vi "FFD.vi"(1 "CK":bool, 2 "Data":bool) -> (0 "Data 2":bool)   [LabVIEW 2012]
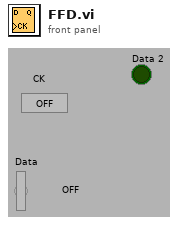
[diagram p1: front panel]
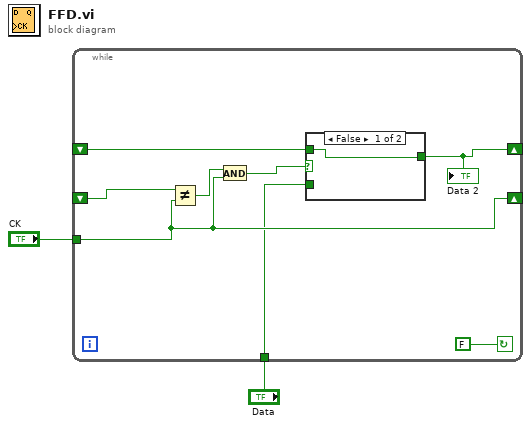
[diagram p0: block diagram]
diagram:
  n1 = while {
    shift-right: [w4] -> _
    shift-left: _ -> [w10]
    shift-right: [w7] -> _
    shift-left: _ -> [w6]
    tunnel: "CK" -> [w4]
    tunnel: "Data" -> [w3]
    stop <- FALSE continue-if-true
    n2 = Not Equal?(x=w10, y=w4) -> (x != y?=w9:bool)
    n3 = And(x=w9, y=w4) -> (x .and. y?=w8:bool)
    n4 = case shown="False" w8 {
      tunnel: w3 -> [_ w12]
      tunnel: [w11 w12] -> w7
      tunnel: w6 -> [w11 _]
      frame False {
      }
      frame True {
      }
    }
    "Data 2" <- w7
  }
